vi "3.vi"() -> ()   [LabVIEW 2020]
panel:
  in  "stop":bool
  out "Waveform\n Graph 2":dynamicdata(graph)
  out "Waveform \nGraph":dynamicdata(graph)
  in  "Phase":dbl
  in  "Amplitude":dbl
  in  "Frequency":dbl
  in  "Offset":dbl
  # "VI Code to display sinusoidal\nand triangular waveforms"
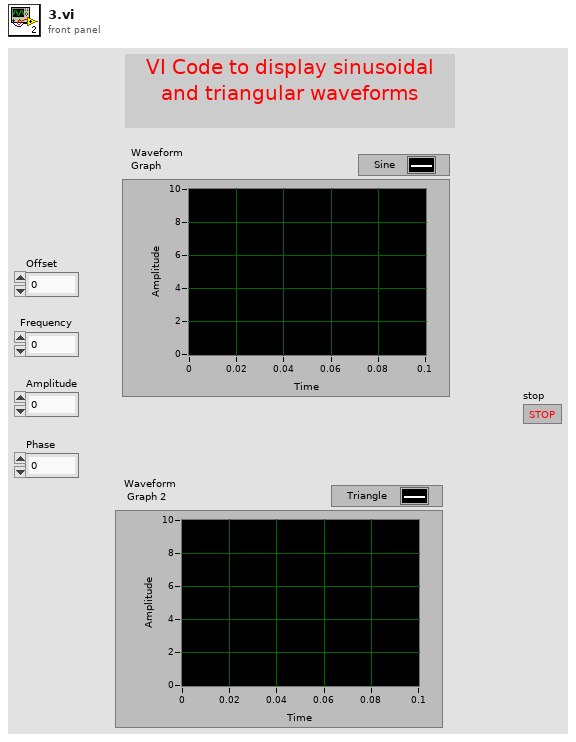
[diagram p1: front panel]
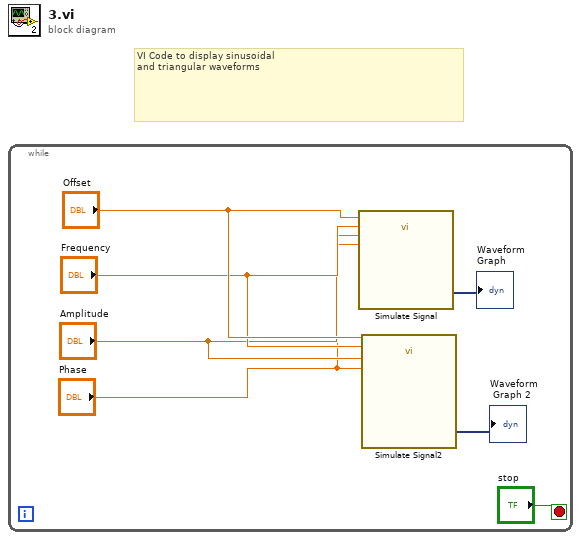
[diagram p0: block diagram]
diagram:
  # "VI Code to display sinusoidal\nand triangular waveforms"
  n1 = while {
    stop <- "stop" stop-if-true
    n2 = call "Simulate Signal"("Offset"="Offset", "Frequency"="Frequency", "Amplitude"="Amplitude", "Phase"="Phase") -> ("Sine"=→"Waveform \nGraph":dynamicdata)  [unwired: 10 in, 1 out]
    n3 = call "Simulate Signal2"("Offset"="Offset", "Frequency"="Frequency", "Amplitude"="Amplitude", "Phase"="Phase") -> ("Triangle"=→"Waveform\n Graph 2":dynamicdata)  [unwired: 10 in, 1 out]
  }
